vi "PYTHON Get Data__ogtk.vi"   [LabVIEW 2017]
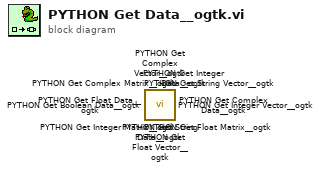
[diagram p0: block diagram]
diagram:
  n1 = call <userlib>:"PYTHON Get String Data__ogtk.vi"() -> ()  [unwired: 5 in, 3 out]
  n2 = call <userlib>:"PYTHON Get Integer Data__ogtk.vi"() -> ()  [unwired: 5 in, 3 out]
  n3 = call <userlib>:"PYTHON Get Float Data__ogtk.vi"() -> ()  [unwired: 5 in, 3 out]
  n4 = call <userlib>:"PYTHON Get Complex Data__ogtk.vi"() -> ()  [unwired: 5 in, 3 out]
  n5 = call <userlib>:"PYTHON Get Complex Matrix__ogtk.vi"() -> ()  [unwired: 5 in, 3 out]
  n6 = call <userlib>:"PYTHON Get Complex Vector__ogtk.vi"() -> ()  [unwired: 5 in, 3 out]
  n7 = call <userlib>:"PYTHON Get Float Matrix__ogtk.vi"() -> ()  [unwired: 5 in, 3 out]
  n8 = call <userlib>:"PYTHON Get Float Vector__ogtk.vi"() -> ()  [unwired: 5 in, 3 out]
  n9 = call <userlib>:"PYTHON Get Integer Matrix__ogtk.vi"() -> ()  [unwired: 5 in, 3 out]
  n10 = call <userlib>:"PYTHON Get Integer Vector__ogtk.vi"() -> ()  [unwired: 5 in, 3 out]
  n11 = call <userlib>:"PYTHON Get Boolean Data__ogtk.vi"() -> ()  [unwired: 5 in, 3 out]
  n12 = call <userlib>:"PYTHON Get String Vector__ogtk.vi"() -> ()  [unwired: 5 in, 3 out]
